vi "test-linear-filter-get-data.vi"(11 "T":dbl) -> (3 "Output":dbl)   [LabVIEW 2019]
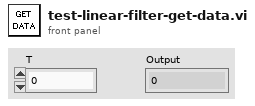
[diagram p1: front panel]
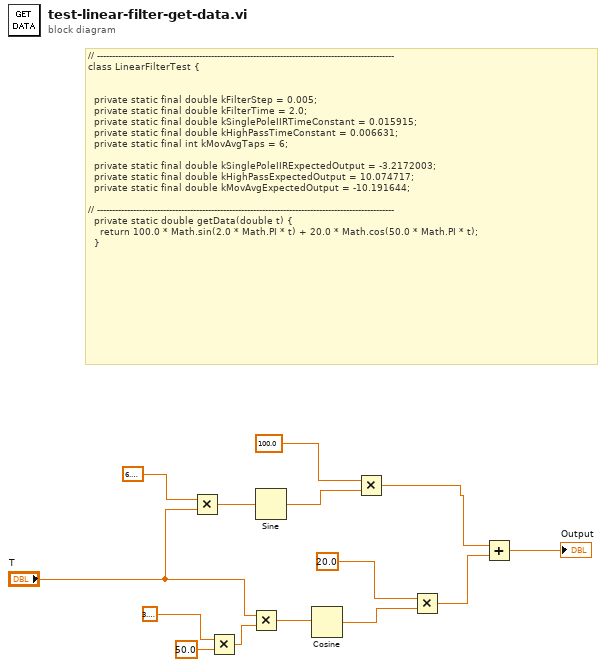
[diagram p0: block diagram]
diagram:
  # "// ---------------------------------------------------------------------------------------------------\nclass LinearFilterTest {\n\n\n  private static final double kFilterStep = 0.005;\n  private static final double kFilterTime = 2.0;\n  private static final double kSinglePoleIIRTimeConstant = 0.015915;\n  private static final double kHighPassTimeConstant = 0.006631;\n  private static final int kMovAvgTaps = 6;\n\n  private static final double kSinglePoleIIRExpectedOutput = -3.2172003;\n  private static final double kHighPassExpectedOutput = 10.074717;\n  private static final double kMovAvgExpectedOutput = -10.191644;\n\n// ---------------------------------------------------------------------------------------------------\n  private static double getData(double t) {\n    return 100.0 * Math.sin(2.0 * Math.PI * t) + 20.0 * Math.cos(50.0 * Math.PI * t);\n  }"
  n1 = Multiply(x=6.283185307179586, y="T") -> (x*y=w11:dbl)
  n2 = Multiply(x=3.141592653589793, y=50.0) -> (x*y=w5:dbl)
  n3 = Multiply(x="T", y=w5) -> (x*y=w6:dbl)
  n4 = Sine(x=w11) -> (sin(x)=w13:dbl)
  n5 = Cosine(x=w6) -> (cos(x)=w9:dbl)
  n6 = Multiply(x=100.0, y=w13) -> (x*y=w3:dbl)
  n7 = Multiply(x=20.0, y=w9) -> (x*y=w2:dbl)
  n8 = Add(x=w3, y=w2) -> (x+y=→"Output":dbl)
